vi "test.video injest payload.vi"() -> ()   [LabVIEW 2020]
uses:
  datasources/video/video.lvclass
  nominal types/timestampManifest/mcap/mcap.lvclass
  nominal types/id/id.lvclass
  datasources/s3/s3.lvclass
  datasources/target/target.lvclass
  <vilib>/JDP Science/JSONtext/JSONtext.lvlib
  nominal types/channelConfig/channelConfig.lvclass
  C:/code/labview-client/lv_src/nominal types/filterTypes/filterTypes.lvclass
  C:/code/labview-client/lv_src/Nominal Client/datasources/payload/payload.lvclass
  C:/code/labview-client/lv_src/nominal types/id/id.lvclass
  C:/code/labview-client/lv_src/Nominal Client/datasources/source/source.lvclass
  C:/code/labview-client/lv_src/Nominal Client/datasources/s3/s3.lvclass
  C:/code/labview-client/lv_src/nominal types/timestampManifest/timestampManifest/timestampManifest.lvclass
  C:/code/labview-client/lv_src/nominal types/timestampManifest/mcap/mcap.lvclass
panel:
  out "<JSON>":string caption="<JSON>First JSON Value"
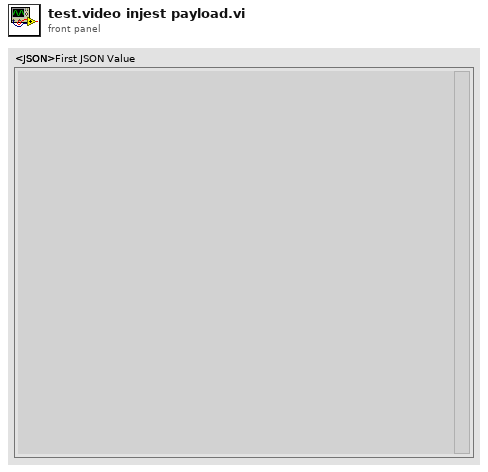
[diagram p1: front panel]
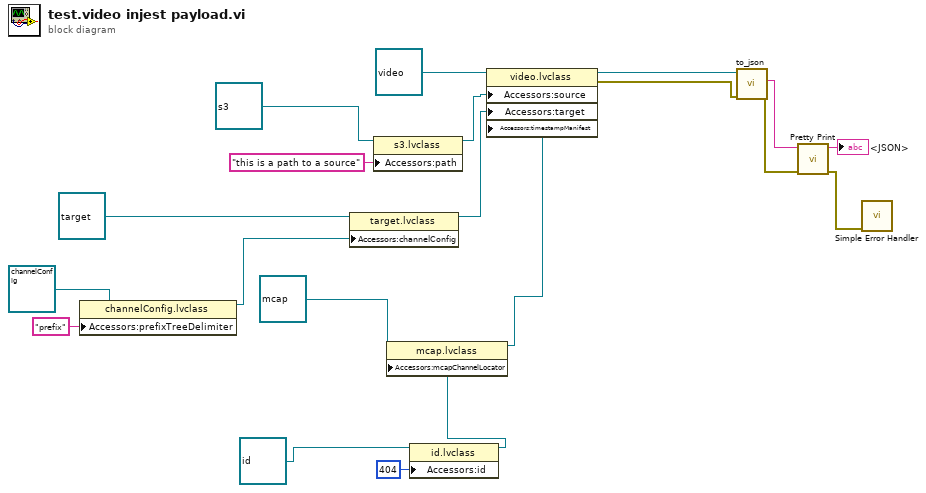
[diagram p0: block diagram]
diagram:
  n1 = property class="channelConfig.lvclass"(reference=refnum<class "channelConfig.lvclass"> refnum ("channelConfig"), "Accessors:prefixTreeDelimiter"="prefix" ("prefixTreeDelimiter")) -> (reference out=w1:refnum<class "channelConfig.lvclass">)  [unwired: 1 in, 1 out]
  n2 = property class="target.lvclass"(reference=refnum<class "target.lvclass"> refnum ("datasources.lvlib:target.lvclass"), "Accessors:channelConfig"=w1) -> (reference out=w10:refnum<class "target.lvclass">)  [unwired: 1 in, 1 out]
  n3 = property class="s3.lvclass"(reference=refnum<class "s3.lvclass"> refnum ("datasources.lvlib:s3.lvclass"), "Accessors:path"="this is a path to a source" ("path")) -> (reference out=w12:refnum<class "s3.lvclass">)  [unwired: 1 in, 1 out]
  n4 = property class="id.lvclass"(reference=refnum<class "id.lvclass"> refnum ("nominal types.lvlib:channelFilter.lvlib:id.lvclass"), "Accessors:id"=404 ("id")) -> (reference out=w15:refnum<class "id.lvclass">)  [unwired: 1 in, 1 out]
  n5 = property class="mcap.lvclass"(reference=refnum<class "mcap.lvclass"> refnum ("nominal types.lvlib:timestampManifest.lvlib:mcap.lvclass"), "Accessors:mcapChannelLocator"=w15) -> (reference out=w17:refnum<class "mcap.lvclass">)  [unwired: 1 in, 1 out]
  n6 = property class="video.lvclass"(reference=refnum<class "video.lvclass"> refnum ("video in"), "Accessors:source"=w12, "Accessors:target"=w10, "Accessors:timestampManifest"=w17) -> (reference out=w19:refnum<class "video.lvclass">, error out=w9:errorcluster)  [unwired: 1 in]
  n7 = call-dynamic "to_json.vi"("error in"=w9, "video in"=w19) -> ("error out"=w6:errorcluster, "json"=w8:string)  [unwired: 6 in, 2 out]
  n8 = call <vilib>:"Pretty Print.vi"("error in (no error)"=w6, "JSON"=w8) -> ("error out"=w5:errorcluster, "<JSON>"=→"<JSON>":string)  [unwired: 7 in, 1 out]
  n9 = call <vilib>:"Simple Error Handler.vi"("error in (no error)"=w5) -> ()  [unwired: 4 in, 5 out]
